vi "mediaIntesecaoCameras_v2.vi"(10 "Field Geometry In":T3, 11 "Cameras Array":T4[](array[typedef]) {"robots_blue"."height" format="%+4.3f"; "robots_blue"."pixel_y" format="%+4.3f"; "robots_blue"."pixel_x" format="%+4.3f"; "robots_blue"."orientation" format="%+4.3f"; "robots_blue"."y" format="%+4.3f"; "robots_blue"."confidence" format="%4.3f"; "robots_blue"."x" format="%+4.3f"; "robots_yellow"."height" format="%+4.3f"; "robots_yellow"."pixel_y" format="%+4.3f"; "robots_yellow"."pixel_x" format="%+4.3f"; "robots_yellow"."orientation" format="%+4.3f"; "robots_yellow"."y" format="%+4.3f"; "robots_yellow"."confidence" format="%4.3f"; "robots_yellow"."x" format="%+4.3f"}) -> (3 "frame out":T4 {"robots_blue"."height" format="%+4.3f"; "robots_blue"."pixel_y" format="%+4.3f"; "robots_blue"."pixel_x" format="%+4.3f"; "robots_blue"."orientation" format="%+4.3f"; "robots_blue"."y" format="%+4.3f"; "robots_blue"."confidence" format="%4.3f"; "robots_blue"."x" format="%+4.3f"; "robots_yellow"."height" format="%+4.3f"; "robots_yellow"."pixel_y" format="%+4.3f"; "robots_yellow"."pixel_x" format="%+4.3f"; "robots_yellow"."orientation" format="%+4.3f"; "robots_yellow"."y" format="%+4.3f"; "robots_yellow"."confidence" format="%4.3f"; "robots_yellow"."x" format="%+4.3f"})   [LabVIEW 2018]
uses:
  SSL Detection Frame.ctl
  SSL Detection Robot.ctl
  <vilib>/Analysis/Matrix/Datatypes/RealMatrix.ctl
  SSL Detection Ball.ctl
  <vilib>/Analysis/Matrix/NI_Matrix.lvlib
panel:
  in  "Array":T1[](array[typedef])
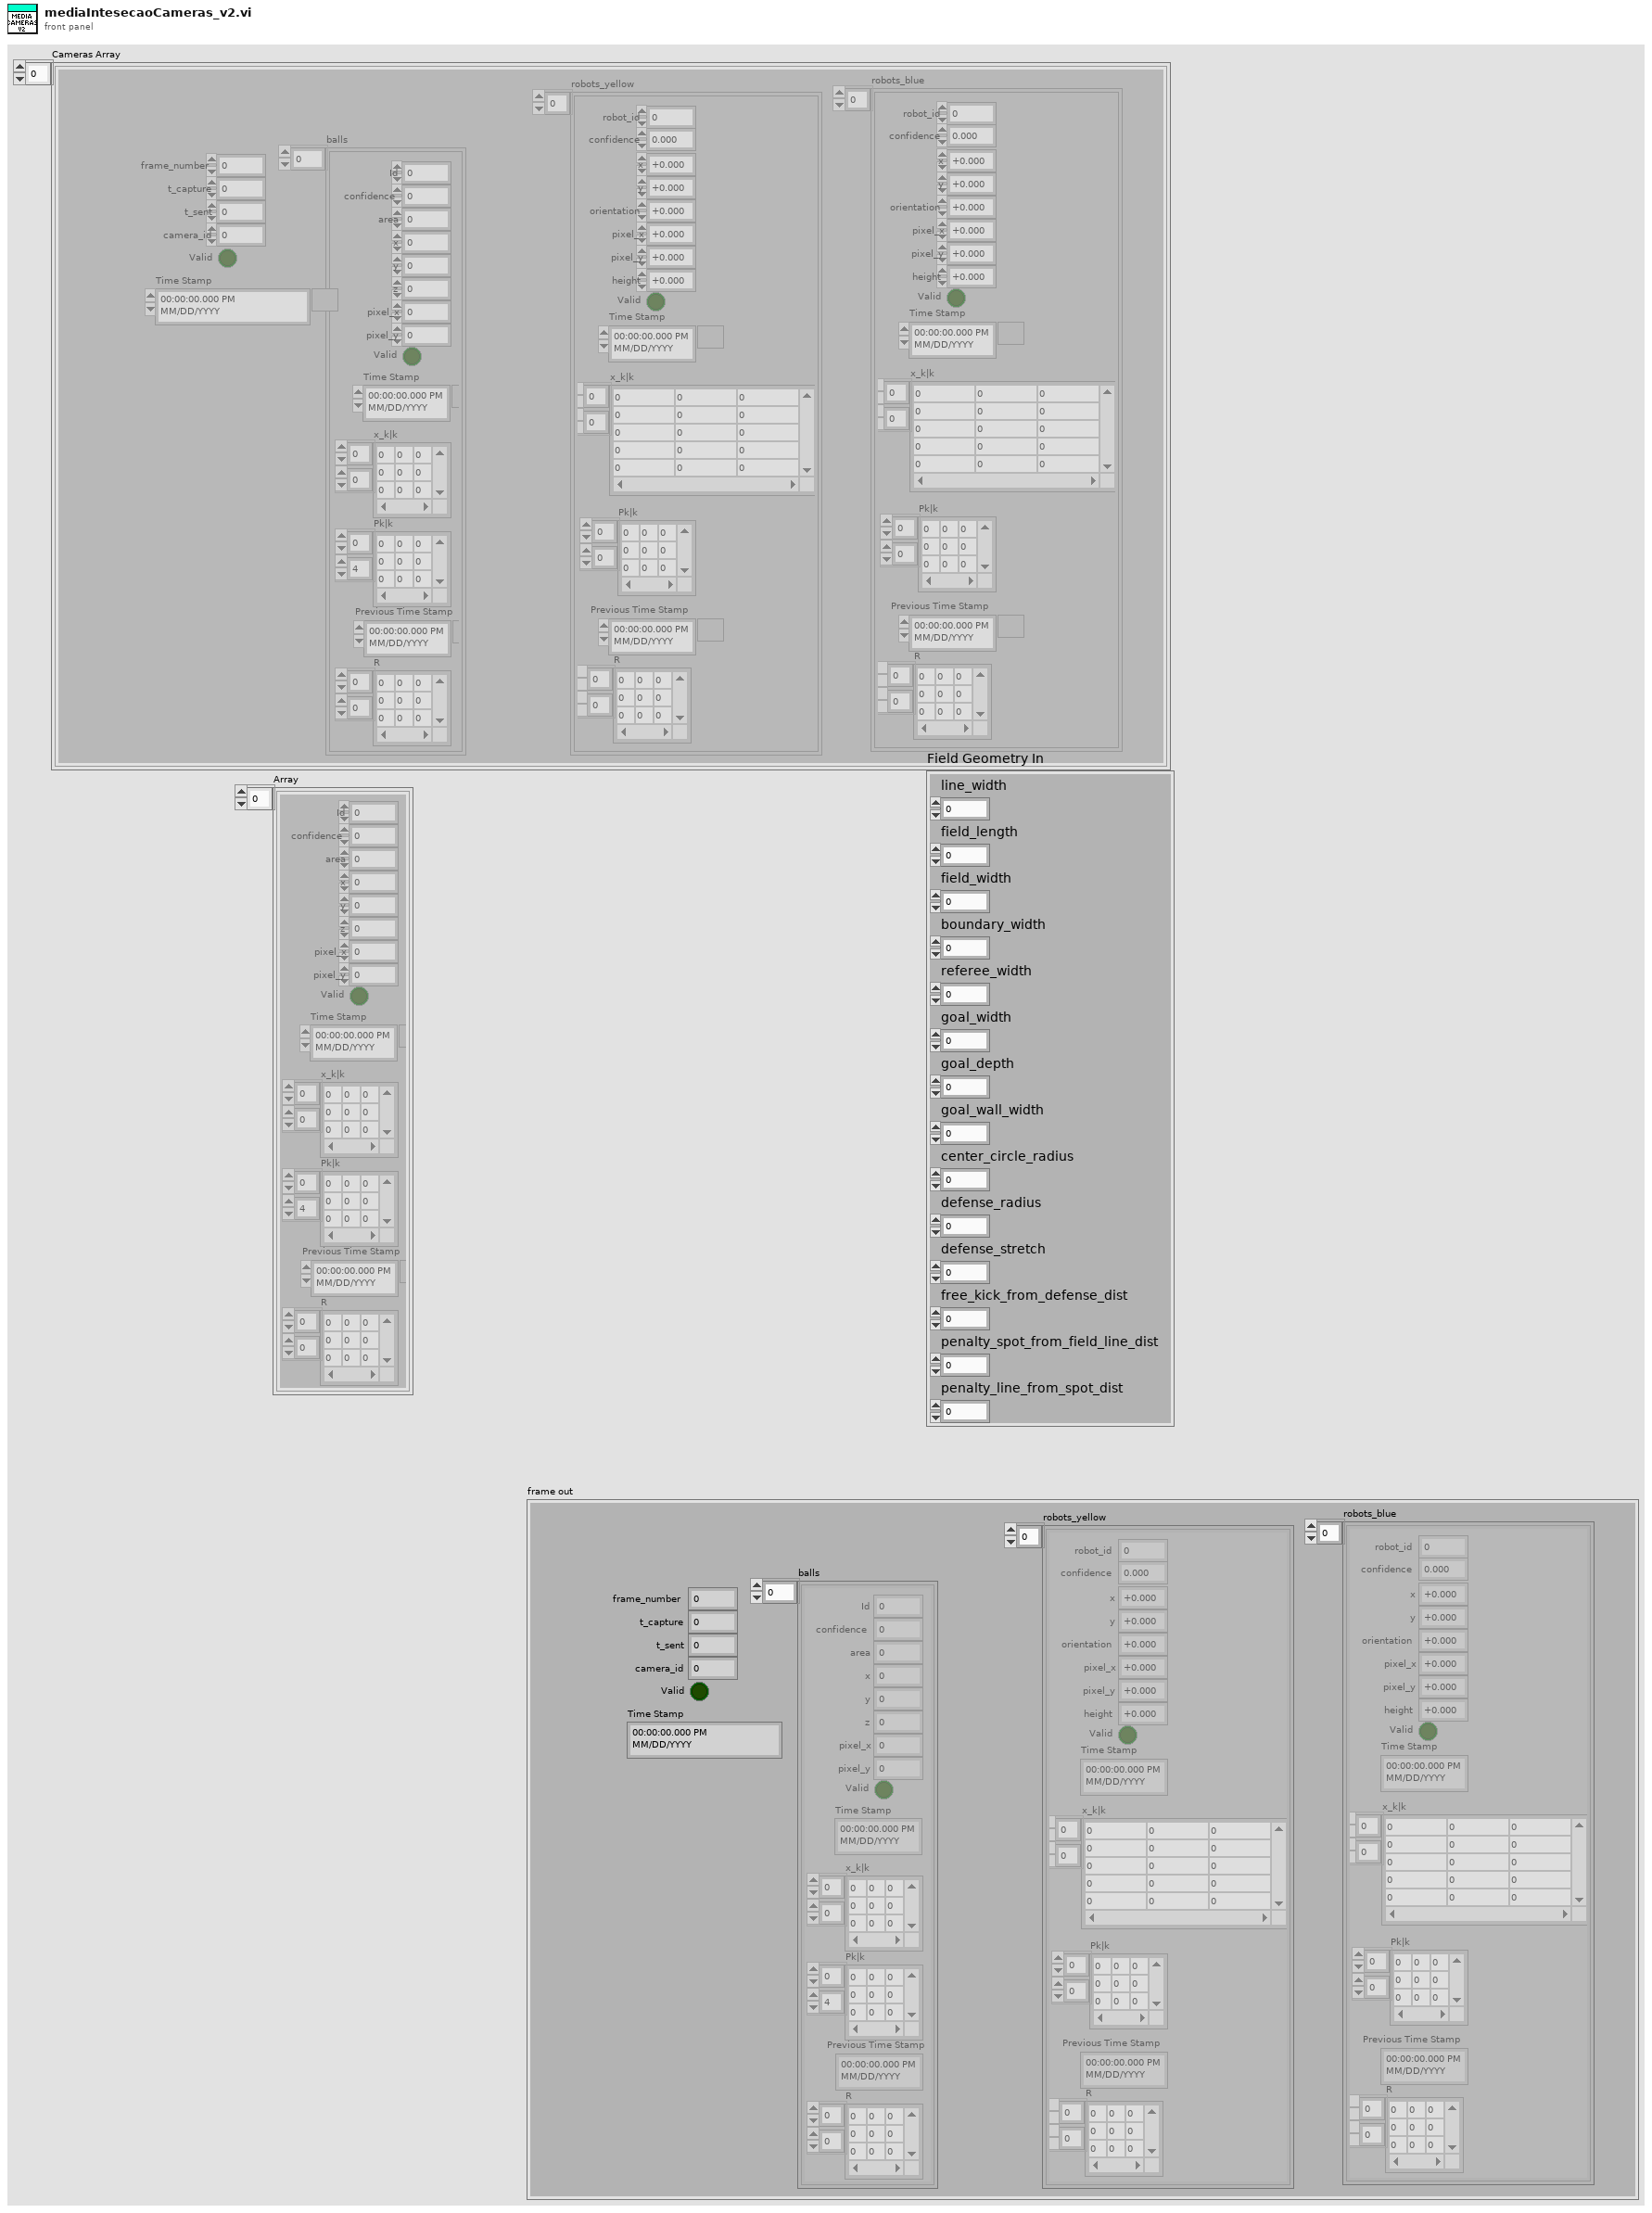
[diagram p1: front panel]
types:
  T1 = typedef "SSL Detection Ball.ctl" = cluster{"x":sgl, "area":u32, "confidence":sgl, "y":sgl, "z":sgl, "pixel_x":sgl, "pixel_y":sgl, "Valid":bool, "Time Stamp":timestamp, "x_k|k":T2, "Pk|k":T2, "Id":u32, "Previous Time Stamp":timestamp, "R":T2}
  T2 = typedef "NI_Matrix.lvlib/RealMatrix.ctl" = dbl[][]
  T3 = cluster{"line_width":u32, "field_length":u32, "field_width":u32, "boundary_width":u32, "referee_width":u32, "goal_width":u32, "goal_depth":u32, "goal_wall_width":u32, "center_circle_radius":u32, "defense_radius":u32, "defense_stretch":u32, "free_kick_from_defense_dist":u32, "penalty_spot_from_field_line_dist":u32, "penalty_line_from_spot_dist":u32}
  T4 = typedef "SSL Detection Frame.ctl" = cluster{"frame_number":u32, "t_capture":dbl, "t_sent":dbl, "camera_id":u32, "robots_yellow":T5[], "robots_blue":T5[], "balls":T1[], "Valid":bool, "Time Stamp":timestamp}
  T5 = typedef "SSL Detection Robot.ctl" = cluster{"x":sgl, "robot_id":u32, "confidence":sgl, "y":sgl, "orientation":sgl, "pixel_x":sgl, "pixel_y":sgl, "height":sgl, "Valid":bool, "Time Stamp":timestamp, "x_k|k":T2, "Pk|k":T2, "Previous Time Stamp":timestamp, "R":T2}
  T6 = cluster{"x":sgl, "y":sgl, "orientation":sgl, "robot_id":u32, "camera_id":u32, "Valid":bool}
  T7 = cluster{"x":sgl, "y":sgl, "camera_id":u32, "Valid":bool}
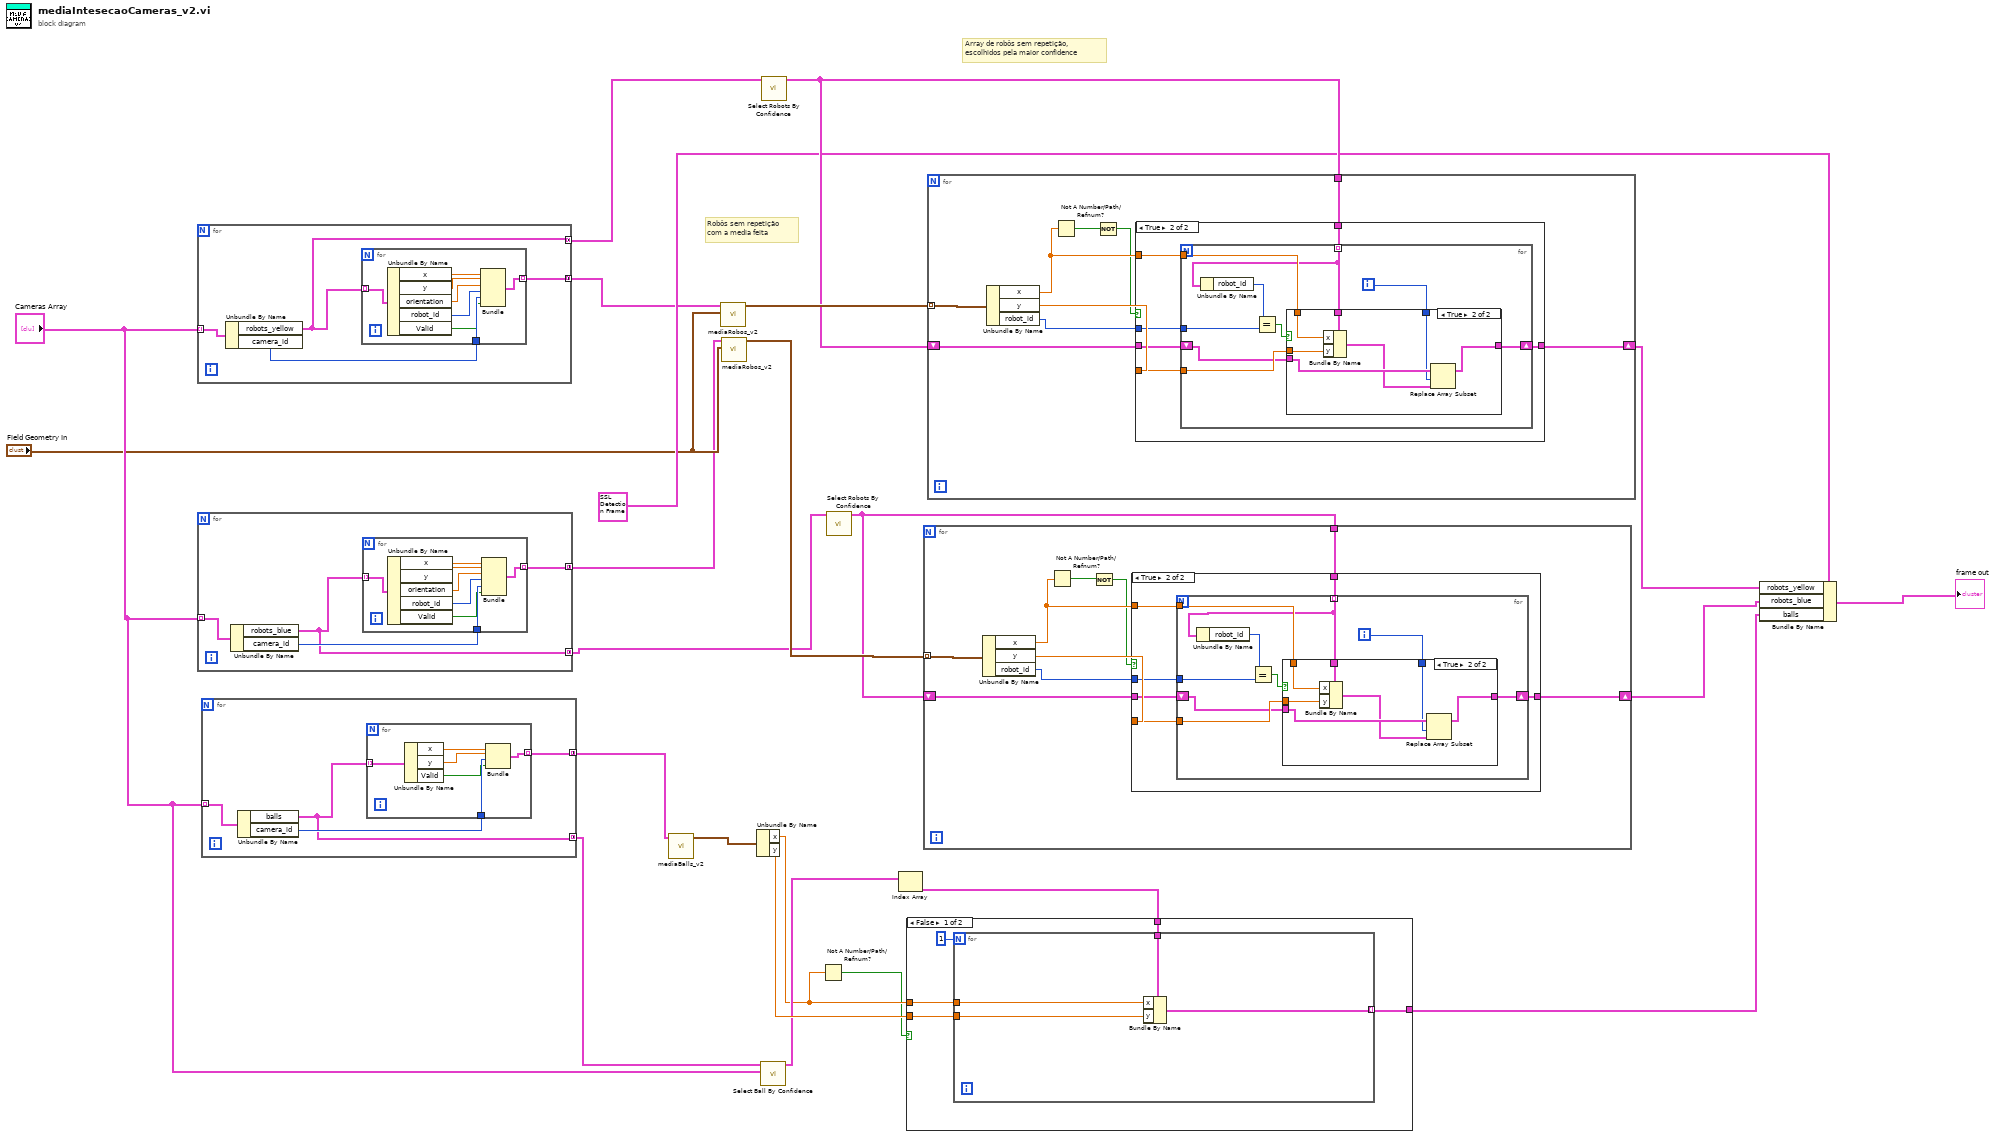
[diagram p0: block diagram]
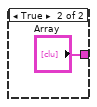
[diagram p2: hidden frame]
diagram:
  # "Robôs sem repetição \ncom a media feita"
  # "Array de robôs sem repetição,\nescolhidos pela maior confidence"
  n1 = for {
    tunnel: "Cameras Array" -> [w27] mode=indexing
    tunnel: [w26] -> w5 mode=concatenating
    tunnel: [w24] -> w19 mode=concatenating
    n2 = Unbundle By Name(w27) -> ("robots_yellow"=w24:T5[], "camera_id"=w25:u32)
    n3 = for {
      tunnel: w24 -> [w35] mode=indexing
      tunnel: [w32] -> w26 mode=indexing
      tunnel: w25 -> [w29]
      n4 = Unbundle By Name(w35) -> ("x"=w34:sgl, "y"=w33:sgl, "orientation"=w31:sgl, "robot_id"=w30:u32, "Valid"=w28:bool)
      n5 = Bundle("x"=w34, "y"=w33, "orientation"=w31, "robot_id"=w30, "camera_id"=w29, "Valid"=w28) -> (w32:T6)  [unwired: 1 in]
    }
  }
  n6 = for {
    tunnel: "Cameras Array" -> [w39] mode=indexing
    tunnel: [w38] -> w4 mode=concatenating
    tunnel: [w36] -> w15 mode=concatenating
    n7 = Unbundle By Name(w39) -> ("robots_blue"=w36:T5[], "camera_id"=w37:u32)
    n8 = for {
      tunnel: w36 -> [w47] mode=indexing
      tunnel: [w44] -> w38 mode=indexing
      tunnel: w37 -> [w41]
      n9 = Unbundle By Name(w47) -> ("x"=w46:sgl, "y"=w45:sgl, "orientation"=w43:sgl, "robot_id"=w42:u32, "Valid"=w40:bool)
      n10 = Bundle("x"=w46, "y"=w45, "orientation"=w43, "robot_id"=w42, "camera_id"=w41, "Valid"=w40) -> (w44:T6)  [unwired: 1 in]
    }
  }
  n11 = for {
    tunnel: "Cameras Array" -> [w51] mode=indexing
    tunnel: [w50] -> w3 mode=concatenating
    tunnel: [w48] -> w12 mode=concatenating
    n12 = Unbundle By Name(w51) -> ("balls"=w48:T1[], "camera_id"=w49:u32)
    n13 = for {
      tunnel: w48 -> [w57] mode=indexing
      tunnel: [w54] -> w50 mode=indexing
      tunnel: w49 -> [w53]
      n14 = Unbundle By Name(w57) -> ("x"=w56:sgl, "y"=w55:sgl, "Valid"=w52:bool)
      n15 = Bundle("x"=w56, "y"=w55, "camera_id"=w53, "Valid"=w52) -> (w54:T7)  [unwired: 1 in]
    }
  }
  n16 = call "mediaBalls_v2.vi"("Array Ball Pose + CamID"=w3) -> ("Ball out"=w21:cluster{"x":dbl, "y":dbl})  [unwired: 10 in]
  n17 = call "mediaRobos_v2.vi"("Field Size 2"="Field Geometry In", "Array Robot Pose + CamID"=w5) -> ("Array"=w23:cluster{"x":dbl, "y":dbl, "robot_id":i32}[])  [unwired: 9 in]
  n18 = call "mediaRobos_v2.vi"("Field Size 2"="Field Geometry In", "Array Robot Pose + CamID"=w4) -> ("Array"=w16:cluster{"x":dbl, "y":dbl, "robot_id":i32}[])  [unwired: 9 in]
  n19 = Unbundle By Name(w21) -> ("x"=w2:dbl, "y"=w20:dbl)
  n20 = call "Select Ball By Confidence.vi"("Array"="Cameras Array", "balls"=w12) -> ("balls out"=w10:T1[])  [unwired: 9 in]
  n21 = call "Select Robots By Confidence.vi"("robots_blue"=w19) -> ("Array"=w18:T5[])  [unwired: 10 in]
  n22 = Not A Number/Path/Refnum?(number/path/refnum=w2) -> (NaN/Path/Refnum?=w1:bool)
  n23 = call "Select Robots By Confidence.vi"("robots_blue"=w15) -> ("Array"=w14:T5[])  [unwired: 10 in]
  n24 = Index Array(array=w10) -> (element=w9:T1)  [unwired: 1 in]
  n25 = case shown="False" w1 {
    tunnel: w20 -> [w62 _]
    tunnel: w9 -> [w61 _]
    tunnel: [w60 "Array"] -> w8
    tunnel: w2 -> [w58 _]
    frame False {
      n26 = for {
        N: 1 -> [_]
        tunnel: w58 -> [w63]
        tunnel: w62 -> [w66]
        tunnel: [w65] -> w60 mode=indexing
        tunnel: w61 -> [w64]
        n27 = Bundle By Name(cluster=w64, "x"=w63, "y"=w66) -> (w65:T1)
      }
    }
    frame True {
    }
  }
  n28 = for {
    tunnel: w16 -> [w76] mode=indexing
    tunnel: w14 -> [w70]
    shift-right: [w74] -> w13
    shift-left: w14 -> [w68]
    n29 = Unbundle By Name(w76) -> ("x"=w73:dbl, "y"=w75:dbl, "robot_id"=w69:i32)
    n30 = Not A Number/Path/Refnum?(number/path/refnum=w73) -> (NaN/Path/Refnum?=w72:bool)
    n31 = Not(x=w72) -> (.not. x?=w71:bool)
    n32 = case shown="True" w71 {
      tunnel: w73 -> [_ w83]
      tunnel: w75 -> [_ w82]
      tunnel: [w77 w81] -> w74
      tunnel: w70 -> [_ w80]
      tunnel: w69 -> [_ w79]
      tunnel: w68 -> [w77 w78]
      frame False {
      }
      frame True {
        n33 = for {
          tunnel: w83 -> [w92]
          tunnel: w82 -> [w91]
          shift-right: [w85] -> w81
          shift-left: w78 -> [w86]
          tunnel: w80 -> [w87] mode=indexing
          tunnel: w79 -> [w89]
          i -> [w84]
          n34 = Unbundle By Name(w87) -> ("robot_id"=w90:u32)
          n35 = Equal?(x=w90, y=w89) -> (x = y?=w88:bool)
          n36 = case shown="True" w88 {
            tunnel: w92 -> [_ w100]
            tunnel: w91 -> [_ w99]
            tunnel: w87 -> [_ w98]
            tunnel: w86 -> [w93 w97]
            tunnel: [w93 w96] -> w85
            tunnel: w84 -> [_ w94]
            frame False {
            }
            frame True {
              n37 = Bundle By Name(cluster=w98, "x"=w100, "y"=w99) -> (w95:T5)
              n38 = Replace Array Subset(array=w97, new element=w95, index=w94) -> (w96:T5[])
            }
          }
        }
      }
    }
  }
  n39 = for {
    tunnel: w23 -> [w109] mode=indexing
    tunnel: w18 -> [w103]
    shift-right: [w107] -> w17
    shift-left: w18 -> [w101]
    n40 = Unbundle By Name(w109) -> ("x"=w106:dbl, "y"=w108:dbl, "robot_id"=w102:i32)
    n41 = Not A Number/Path/Refnum?(number/path/refnum=w106) -> (NaN/Path/Refnum?=w105:bool)
    n42 = Not(x=w105) -> (.not. x?=w104:bool)
    n43 = case shown="True" w104 {
      tunnel: w106 -> [_ w116]
      tunnel: w108 -> [_ w115]
      tunnel: [w110 w114] -> w107
      tunnel: w103 -> [_ w113]
      tunnel: w102 -> [_ w112]
      tunnel: w101 -> [w110 w111]
      frame False {
      }
      frame True {
        n44 = for {
          tunnel: w116 -> [w125]
          tunnel: w115 -> [w124]
          shift-right: [w118] -> w114
          shift-left: w111 -> [w119]
          tunnel: w113 -> [w120] mode=indexing
          tunnel: w112 -> [w122]
          i -> [w117]
          n45 = Unbundle By Name(w120) -> ("robot_id"=w123:u32)
          n46 = Equal?(x=w123, y=w122) -> (x = y?=w121:bool)
          n47 = case shown="True" w121 {
            tunnel: w125 -> [_ w133]
            tunnel: w124 -> [_ w132]
            tunnel: w120 -> [_ w131]
            tunnel: w119 -> [w126 w130]
            tunnel: [w126 w129] -> w118
            tunnel: w117 -> [_ w127]
            frame False {
            }
            frame True {
              n48 = Bundle By Name(cluster=w131, "x"=w133, "y"=w132) -> (w128:T5)
              n49 = Replace Array Subset(array=w130, new element=w128, index=w127) -> (w129:T5[])
            }
          }
        }
      }
    }
  }
  n50 = Bundle By Name(cluster=T4 {"frame_number"=0, "t_capture"=0.0, "t_sent"=0.0, "camera_id"=0, "robots_yellow"=[], "robots_blue"=[], "balls"=[], "Valid"=TRUE, "Time Stamp"=timestamp(0 s since 1904-01-01)} ("Unico frame"), "robots_yellow"=w17, "robots_blue"=w13, "balls"=w8) -> (→"frame out":T4)
